vi "String to Connection.vi"(11 "String":string) -> (3 "Connection":T1)   [LabVIEW 2017, in "SLSC Switch Scripting.lvlib"]
uses:
  SLSC Switch Scripting.lvlib
  Routing Channel/Connection.ctl
  <vilib>/regexp/Match Regular Expression.xnode
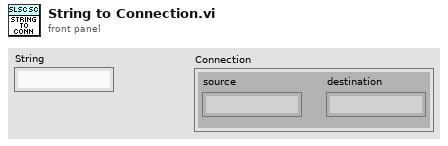
[diagram p1: front panel]
types:
  T1 = typedef "SLSC Switch Scripting.lvlib/Connection.ctl" = cluster{"source":string, "destination":string}
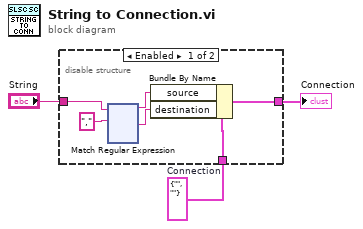
[diagram p0: block diagram]
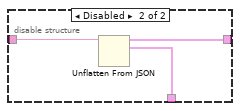
[diagram p2: hidden frame]
diagram:
  w1 = T1 {"source"="", "destination"=""}  # Connection
  n1 = disable-structure shown="Enabled" {
    disable-tunnel: "String" -> [w6 w125]
    disable-tunnel: [w5 w124] -> w2
    disable-tunnel: w1 -> [w4 w126]
    frame Enabled {
      n2 = xnode "Match Regular Expression"("input string"=w6, "regular expression"="," ("search string")) -> ("before match"=w8:string, "after match"=w7:string)  [unwired: 4 in, 3 out]
      n3 = Bundle By Name(cluster=w4, "source"=w8, "destination"=w7) -> (w5:T1)
    }
    frame Disabled {
      n4 = Unflatten From JSON(JSON string=w125, type and defaults=w126) -> (value=w124:T1)  [unwired: 5 in, 1 out]
    }
  }
  "Connection" <- w2
